vi "9-5 2진파일로부터읽기.vi"() -> ()   [LabVIEW 2014]
panel:
  out "error out":errorcluster caption="에러 출력"
  in  "카운트(1)":i32
  in  "오프셋(바이트) (0)":i64=1024
  out "웨이브폼 그래프":dbl[](graph)
  in  "파일 경로(대화 상자 사용)":path=path "C:/Users/LVEDU09/Documents/YSK/2019-03-08/샘플 000.txt"
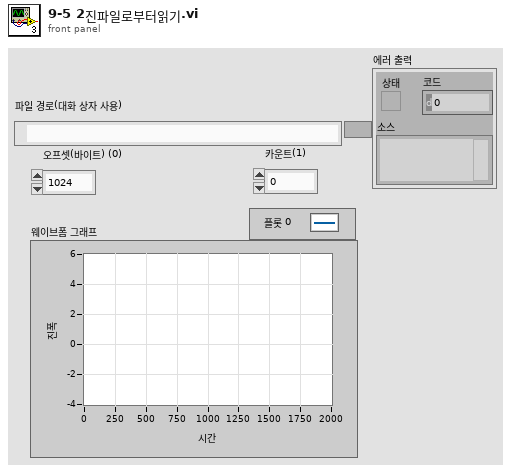
[diagram p1: front panel]
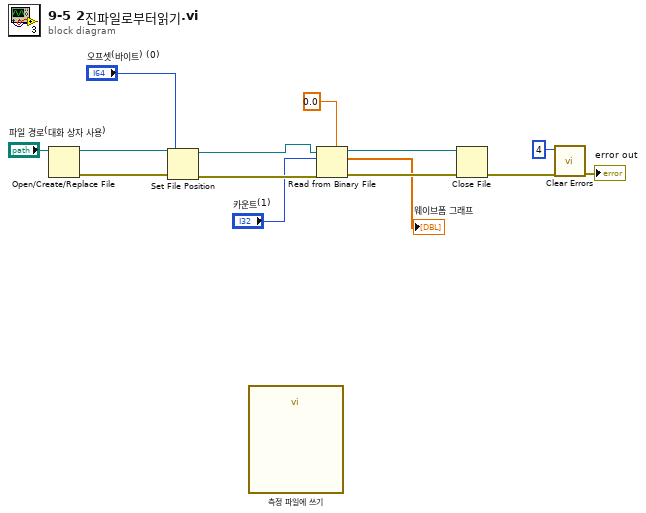
[diagram p0: block diagram]
diagram:
  n1 = Open/Create/Replace File(file path (use dialog)="파일 경로(대화 상자 사용)") -> (refnum out=w9:refnum<file>, error out=w8:errorcluster)  [unwired: 5 in, 1 out]
  n2 = Set File Position(offset (in bytes) (0)="오프셋(바이트) (0)", refnum=w9, error in=w8) -> (refnum out=w6:refnum<file>, error out=w7:errorcluster)  [unwired: 1 in]
  n3 = call "측정 파일에 쓰기"() -> ()  [unwired: 17 in, 3 out]
  n4 = Read from Binary File(5:0.0, 8:w7, 10:"카운트(1)", 11:w6) -> (0:w13:errorcluster, 2:→"웨이브폼 그래프":dbl[], 3:w14:refnum<file>)  [unwired: 2 in, 1 out]
  n5 = Close File(refnum=w14, error in=w13) -> (error out=w3:errorcluster)  [unwired: 1 out]
  n6 = call <vilib>:"Clear Errors.vi"("error in (no error)"=w3, "specific error code to clear (0: all)"=4) -> ("error out"=→"error out":errorcluster)  [unwired: 4 in, 1 out]
